vi "Read Measurement Statistics1.vi"(0 "VISA resource name":refnum<visa-resource-name>, 11 "error in (no error)":errorcluster) -> (2 "Standard Deviation":dbl, 3 "Minimum Value":dbl, 4 "VISA resource name out":refnum<visa-resource-name>, 6 "Arithmetic Mean":dbl, 8 "Measurement Count":dbl, 10 "Maximum Value":dbl, 14 "Peak-to-peak Value":dbl, 15 "error out":errorcluster)   [LabVIEW 2015, in "Agilent 3446X Series1.lvlib"]
doc: "Reads the measurement statistics."
uses:
  Agilent 3446X Series1.lvlib
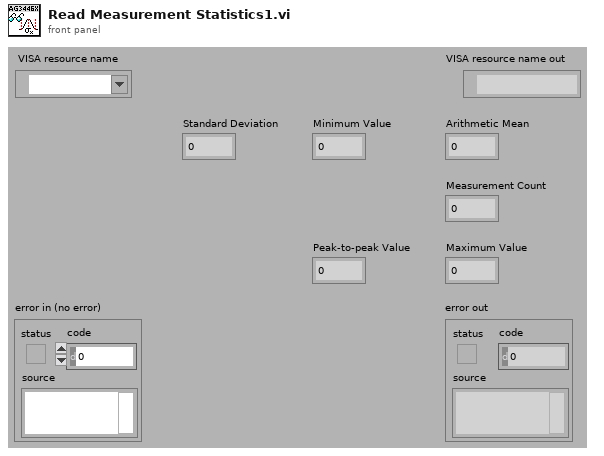
[diagram p1: front panel]
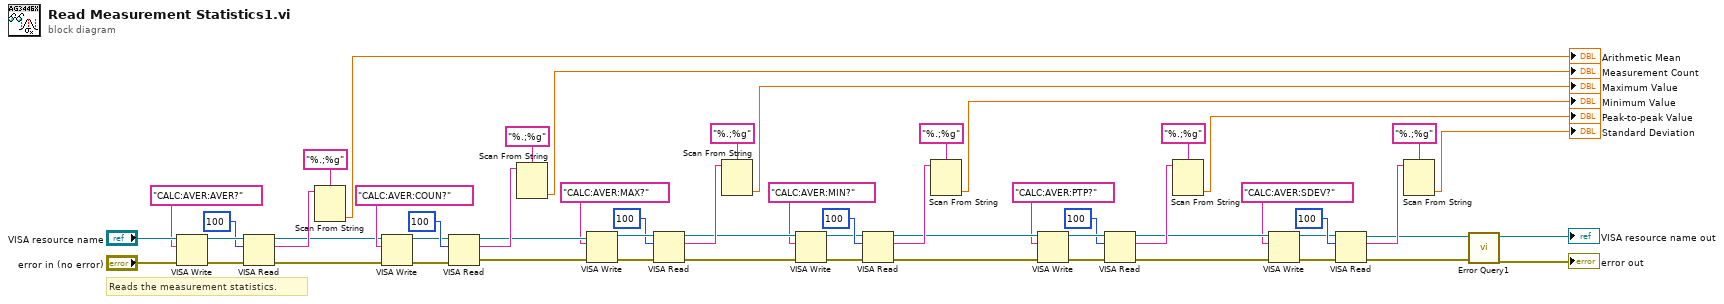
[diagram p0: block diagram]
diagram:
  # "Reads the measurement statistics."
  n1 = VISA Write(VISA resource name="VISA resource name", write buffer="CALC:AVER:AVER?", error in (no error)="error in (no error)") -> (VISA resource name out=w52:refnum<visa-resource-name>, error out=w53:errorcluster)  [unwired: 1 out]
  n2 = VISA Read(VISA resource name=w52, byte count=u32 100, error in (no error)=w53) -> (VISA resource name out=w43:refnum<visa-resource-name>, read buffer=w50:string, error out=w42:errorcluster)  [unwired: 1 out]
  n3 = Scan From String(format string="%.;%g", input string=w50) -> (output 1=→"Arithmetic Mean":dbl)  [unwired: 2 in, 4 out]
  n4 = VISA Write(VISA resource name=w43, write buffer="CALC:AVER:COUN?", error in (no error)=w42) -> (VISA resource name out=w45:refnum<visa-resource-name>, error out=w23:errorcluster)  [unwired: 1 out]
  n5 = VISA Read(VISA resource name=w45, byte count=u32 100, error in (no error)=w23) -> (VISA resource name out=w25:refnum<visa-resource-name>, read buffer=w47:string, error out=w24:errorcluster)  [unwired: 1 out]
  n6 = Scan From String(format string="%.;%g", input string=w47) -> (output 1=→"Measurement Count":dbl)  [unwired: 2 in, 4 out]
  n7 = VISA Write(VISA resource name=w25, write buffer="CALC:AVER:MAX?", error in (no error)=w24) -> (VISA resource name out=w41:refnum<visa-resource-name>, error out=w22:errorcluster)  [unwired: 1 out]
  n8 = VISA Read(VISA resource name=w41, byte count=u32 100, error in (no error)=w22) -> (VISA resource name out=w21:refnum<visa-resource-name>, read buffer=w39:string, error out=w20:errorcluster)  [unwired: 1 out]
  n9 = Scan From String(format string="%.;%g", input string=w39) -> (output 1=→"Maximum Value":dbl)  [unwired: 2 in, 4 out]
  n10 = VISA Write(VISA resource name=w21, write buffer="CALC:AVER:MIN?", error in (no error)=w20) -> (VISA resource name out=w34:refnum<visa-resource-name>, error out=w19:errorcluster)  [unwired: 1 out]
  n11 = VISA Read(VISA resource name=w34, byte count=u32 100, error in (no error)=w19) -> (VISA resource name out=w17:refnum<visa-resource-name>, read buffer=w36:string, error out=w18:errorcluster)  [unwired: 1 out]
  n12 = Scan From String(format string="%.;%g", input string=w36) -> (output 1=→"Minimum Value":dbl)  [unwired: 2 in, 4 out]
  n13 = VISA Write(VISA resource name=w17, write buffer="CALC:AVER:PTP?", error in (no error)=w18) -> (VISA resource name out=w33:refnum<visa-resource-name>, error out=w16:errorcluster)  [unwired: 1 out]
  n14 = VISA Read(VISA resource name=w33, byte count=u32 100, error in (no error)=w16) -> (VISA resource name out=w15:refnum<visa-resource-name>, read buffer=w31:string, error out=w14:errorcluster)  [unwired: 1 out]
  n15 = Scan From String(format string="%.;%g", input string=w31) -> (output 1=→"Peak-to-peak Value":dbl)  [unwired: 2 in, 4 out]
  n16 = VISA Write(VISA resource name=w15, write buffer="CALC:AVER:SDEV?", error in (no error)=w14) -> (VISA resource name out=w26:refnum<visa-resource-name>, error out=w13:errorcluster)  [unwired: 1 out]
  n17 = VISA Read(VISA resource name=w26, byte count=u32 100, error in (no error)=w13) -> (VISA resource name out=w12:refnum<visa-resource-name>, read buffer=w28:string, error out=w11:errorcluster)  [unwired: 1 out]
  n18 = Scan From String(format string="%.;%g", input string=w28) -> (output 1=→"Standard Deviation":dbl)  [unwired: 2 in, 4 out]
  n19 = call "Error Query1.vi"("error in (no error)"=w11, "VISA resource name"=w12) -> ("error out"=→"error out":errorcluster, "VISA resource name out"=→"VISA resource name out":refnum<visa-resource-name>)  [unwired: 8 out]
